vi "LtaExample.vi"() -> ()   [LabVIEW 2018]
uses:
  Comms_lib/CommsData.ctl
  <extravilib>/ChannelInstances/Tag-bool/Write With Abort.vi
  <extravilib>/ChannelInstances/Tag-bool/Read With Abort.vi
  <extravilib>/ChannelInstances/Tag-bool/Instantiate.vi
  <extravilib>/ChannelInstances/Tag-bool/EndpointRead.vi
  <vilib>/Utility/error.llb/Error Cluster From Error Code.vi
  <extravilib>/ChannelInstances/Tag-bool/Endpoint.vi
  <vilib>/ErrorRing/Error Ring.xnode
  Comms_lib/Comms.lvlib
  <extravilib>/ChannelInstances/Tag-bool.lvlib
  LV-PY_Lib/LV-PY.lvlib
panel:
  in  "MyCluster":T1
  out "Enum Out":enum16{"Foo", "Bar", "Do", "Rey", "Mi"}(ring)
  in  "btnRun":bool
  out "D":dbl
  in  "C":dbl=1.0
  in  "B":dbl=1.0
  in  "A":dbl=1.0
  in  "btnPlay":bool
  in  "Script":path=path "X:/Projects/PMUCal/LV_TestAutomation/Examples/example.py"
  out "Accepted?":bool
  in  "btnStop":bool
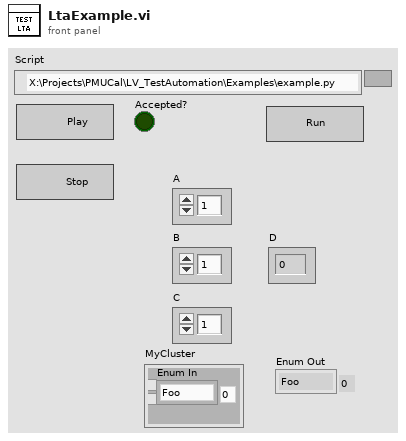
[diagram p1: front panel]
types:
  T1 = cluster{"Enum In":enum16{"Foo", "Bar", "Do", "Rey", "Mi"}}
  T2 = typedef "Comms.lvlib/CommsData.ctl" = cluster{"Command":string, "XMLData":string}
  T3 = typedef "Tag-bool.lvlib/))Channel.ctl" = refnum<queue>
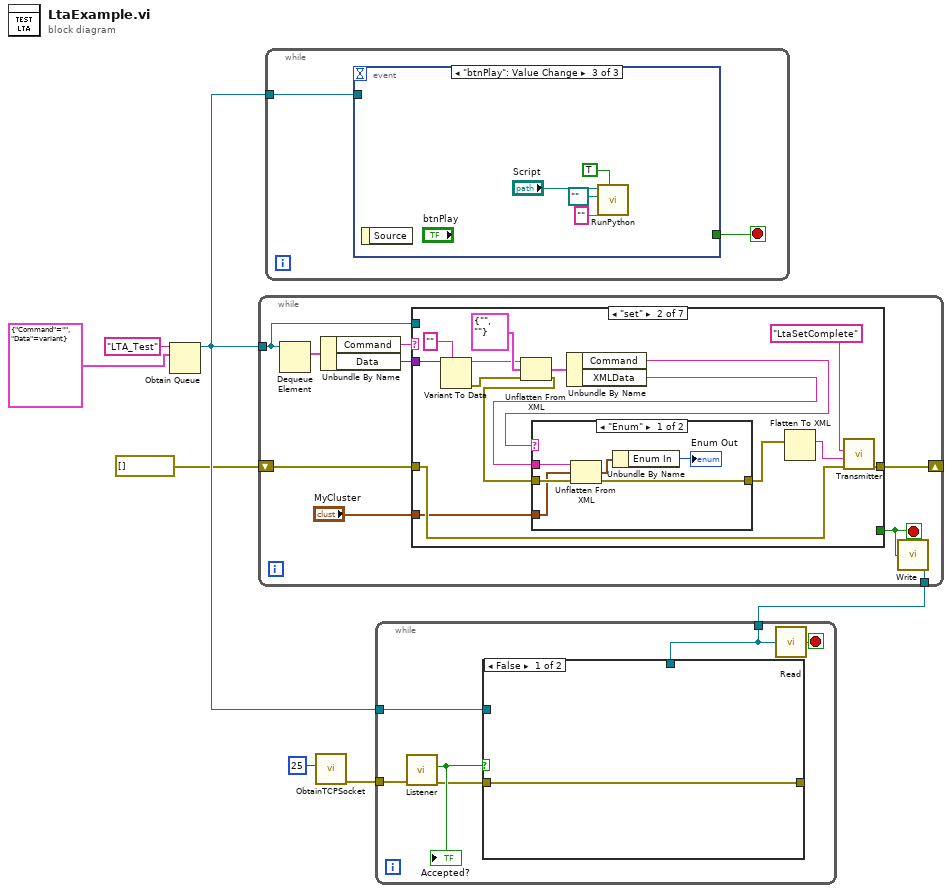
[diagram p0: block diagram]
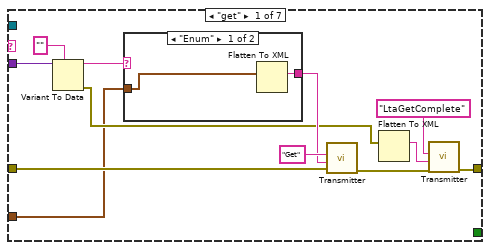
[diagram p2: hidden frame]
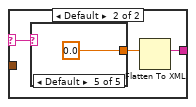
[diagram p3: hidden frame]
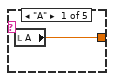
[diagram p4: hidden frame]
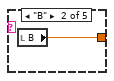
[diagram p5: hidden frame]
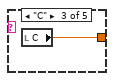
[diagram p6: hidden frame]
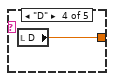
[diagram p7: hidden frame]
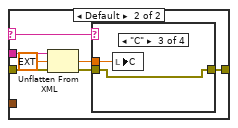
[diagram p8: hidden frame]
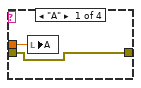
[diagram p9: hidden frame]
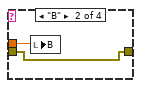
[diagram p10: hidden frame]
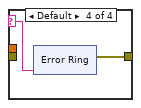
[diagram p11: hidden frame]
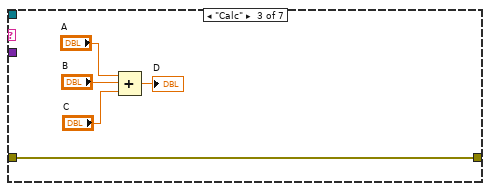
[diagram p12: hidden frame]
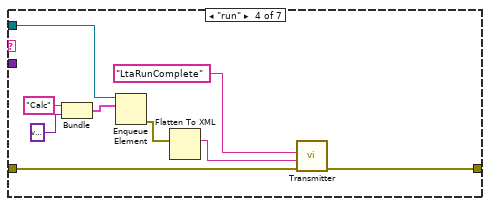
[diagram p13: hidden frame]
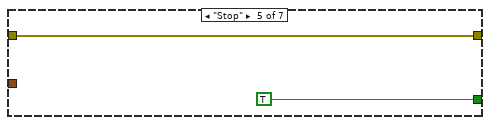
[diagram p14: hidden frame]
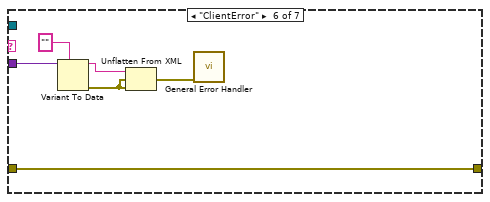
[diagram p15: hidden frame]
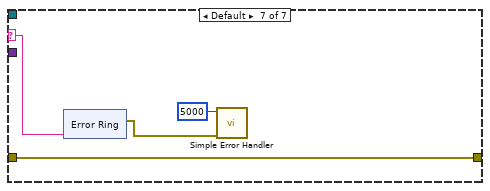
[diagram p16: hidden frame]
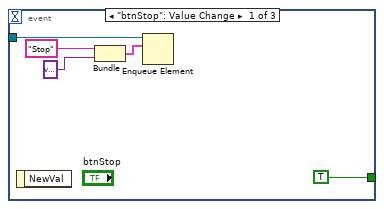
[diagram p17: hidden frame]
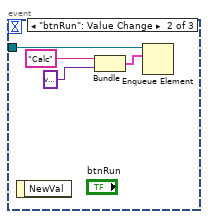
[diagram p18: hidden frame]
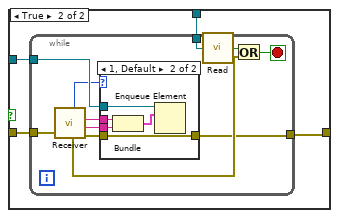
[diagram p19: hidden frame]
diagram:
  n1 = Obtain Queue(name (unnamed)="LTA_Test", element data type=cluster{"Command":string, "Data":variant} {"Command"="", "Data"=variant}) -> (queue out=w2:refnum<queue>)  [unwired: 3 in, 2 out]
  n2 = while {
    tunnel: [w12] -> w5
    tunnel: w2 -> [w11]
    shift-right: [w10] -> _
    shift-left: errorcluster[] [] ("ErrorArray") -> [w9]
    stop <- w13 stop-if-true
    n3 = Dequeue Element(queue=w11) -> (element=w16:cluster{"Command":string, "Data":variant})  [unwired: 2 in, 3 out]
    n4 = Unbundle By Name(w16) -> ("Command"=w15:string, "Data"=w14:variant)
    n5 = case shown="\"set\"" w15 {
      selector: w15 -> [_ _ _ _ _ _ w106]
      tunnel: w14 -> [w28 w53 _ _ _ w103 _]
      tunnel: [_ _ _ _ TRUE _ _] -> w13
      tunnel: w11 -> [_ _ _ w95 _ _ _]
      tunnel: [w22 w51 w82 w91 w96 w98 w104] -> w10
      tunnel: w9 -> [w24 w40 w82 w90 w96 w98 w104]
      tunnel: "MyCluster" -> [w17 w39 _ _ _ _ _]
      frame "get" {
        n6 = Variant To Data(type="", Variant=w28) -> (data=w26:string, error out=w19:errorcluster)  [unwired: 1 in]
        n7 = case shown="\"Enum\"" w26 {
          selector: w26 -> [_ w33]
          tunnel: [w30 w31] -> w20
          tunnel: w17 -> [w29 _]
          frame "Enum" {
            n8 = Flatten To XML(anything=w29) -> (xml string=w30:string)
          }
          frame Default {
            n9 = case shown="Default" w33 {
              tunnel: [w34 w35 w36 w37 0.0 ("D")] -> w32
              frame "A" {
                n10 = local read "A"() -> (w34:dbl)
              }
              frame "B" {
                n11 = local read "B"() -> (w35:dbl)
              }
              frame "C" {
                n12 = local read "C"() -> (w36:dbl)
              }
              frame "D" {
                n13 = local read "D"() -> (w37:dbl)
              }
              frame Default {
              }
            }
            n14 = Flatten To XML(anything=w32) -> (xml string=w31:string)
          }
        }
        n15 = call "Transmitter.vi"("ErrorArray"=w24, "XMLData"=w20, "Command"="Get") -> ("ErrorArray"=w23:errorcluster[])  [unwired: 7 in, 1 out]
        n16 = Flatten To XML(anything=w19) -> (xml string=w18:string)
        n17 = call "Transmitter.vi"("ErrorArray"=w23, "XMLData"=w18, "Command"="LtaGetComplete") -> ("ErrorArray"=w22:errorcluster[])  [unwired: 7 in, 1 out]
      }
      frame "set" {
        n18 = Variant To Data(type="", Variant=w53) -> (data=w47:string, error out=w46:errorcluster)  [unwired: 1 in]
        n19 = Unflatten From XML(xml string=w47, type=T2 {"Command"="", "XMLData"=""} ("CommsData"), error in (no error)=w46) -> (value=w45:T2, error out=w42:errorcluster)
        n20 = Unbundle By Name(w45) -> ("Command"=w44:string, "XMLData"=w43:string)
        n21 = case shown="\"Enum\"" w44 {
          selector: w44 -> [_ w65]
          tunnel: w43 -> [w59 w64]
          tunnel: w42 -> [w58 w63]
          tunnel: [w57 w60] -> w41
          tunnel: w39 -> [w56 _]
          frame "Enum" {
            n22 = Unflatten From XML(xml string=w59, type=w56, error in (no error)=w58) -> (value=w55:T1, error out=w57:errorcluster)
            n23 = Unbundle By Name(w55) -> ("Enum In"=→"Enum Out":enum16{"Foo", "Bar", "Do", "Rey", "Mi"})
          }
          frame Default {
            n24 = Unflatten From XML(xml string=w64, type=ext 0.0 ("D"), error in (no error)=w63) -> (value=w62:ext, error out=w61:errorcluster)
            n25 = case shown="\"C\"" w65 {
              selector: w65 -> [_ _ _ w74]
              tunnel: w62 -> [w68 w70 w72 _]
              tunnel: w61 -> [w67 w69 w71 _]
              tunnel: [w67 w69 w71 w73] -> w60
              frame "A" {
                n26 = local write "A"(w68) -> ()
              }
              frame "B" {
                n27 = local write "B"(w70) -> ()
              }
              frame "C" {
                n28 = local write "C"(w72) -> ()
              }
              frame Default {
                n29 = xnode ("Error Ring")("parameter 0"=w74) -> ("error out"=w73:errorcluster)
              }
            }
          }
        }
        n30 = Flatten To XML(anything=w41) -> (xml string=w49:string)
        n31 = call "Transmitter.vi"("ErrorArray"=w40, "XMLData"=w49, "Command"="LtaSetComplete") -> ("ErrorArray"=w51:errorcluster[])  [unwired: 7 in, 1 out]
      }
      frame "Calc" {
        n32 = Compound Arithmetic op=ADD("A", "B", "C") -> (→"D":dbl)
      }
      frame "run" {
        n33 = Bundle("Calc", variant) -> (w94:cluster{string, variant})  [unwired: 1 in]
        n34 = Enqueue Element(queue=w95, element=w94) -> (error out=w88:errorcluster)  [unwired: 2 in, 2 out]
        n35 = Flatten To XML(anything=w88) -> (xml string=w89:string)
        n36 = call "Transmitter.vi"("ErrorArray"=w90, "XMLData"=w89, "Command"="LtaRunComplete") -> ("ErrorArray"=w91:errorcluster[])  [unwired: 7 in, 1 out]
      }
      frame "Stop" {
      }
      frame "ClientError" {
        n37 = Variant To Data(type="", Variant=w103) -> (data=w100:string, error out=w101:errorcluster)  [unwired: 1 in]
        n38 = Unflatten From XML(xml string=w100, type=w101, error in (no error)=w101) -> (value=w99:errorcluster)  [unwired: 1 out]
        n39 = call <vilib>:"General Error Handler.vi"("error in (no error)"=w99) -> ()  [unwired: 10 in, 5 out]
      }
      frame Default {
        n40 = xnode "Error Ring"("parameter 0"=w106) -> ("error out"=w105:errorcluster)
        n41 = call <vilib>:"Simple Error Handler.vi"("error code (no error:0)"=5000, "error in (no error)"=w105) -> ()  [unwired: 3 in, 5 out]
      }
    }
    n42 = call <extravilib>:"Write.vi"("element"=w13) -> ("channel"=w12:T3)  [unwired: 1 out]
  }
  n43 = while {
    tunnel: w2 -> [w115]
    stop <- w116 stop-if-true
    n44 = event shown="[2] \"btnPlay\": Value Change" {
      selector: _ -> [_ _ _]
      dyn-events: _ -> [_ _ _]
      timeout: _ -> [_ _ _]
      tunnel: [TRUE _ _] -> w116
      tunnel: w115 -> [w120 w125 _]
      event "btnStop": Value Change {
        n45 = event-data() -> ()  [unwired: 1 in, 1 out]
        n46 = Bundle("Stop", variant) -> (w119:cluster{string, variant})  [unwired: 1 in]
        n47 = Enqueue Element(queue=w120, element=w119) -> ()  [unwired: 2 in, 3 out]
      }
      event "btnRun": Value Change {
        n48 = event-data() -> ()  [unwired: 1 in, 1 out]
        n49 = Bundle("Calc", variant) -> (w124:cluster{string, variant})  [unwired: 1 in]
        n50 = Enqueue Element(queue=w125, element=w124) -> ()  [unwired: 2 in, 3 out]
      }
      event "btnPlay": Value Change {
        n51 = event-data() -> ()  [unwired: 1 in, 1 out]
        n52 = call "RunPython.vi"("PathToScript"="Script", "PathToUserDir"=path "", "ScriptDir"="", "keep cmd window open (f)"=TRUE) -> ()  [unwired: 5 in, 2 out]
      }
    }
  }
  n53 = call "ObtainTCPSocket.vi"("timeout"=25) -> ("ErrorArray"=w6:errorcluster[])  [unwired: 9 in, 1 out]
  n54 = while {
    tunnel: w6 -> [w135]
    tunnel: w5 -> [w131]
    tunnel: w2 -> [w130]
    stop <- w134 stop-if-true
    n55 = call "Listener.vi"("ErrorArray"=w135) -> ("ErrorArray"=w132:errorcluster[], "Accepted?"=w133:bool)  [unwired: 9 in]
    "Accepted?" <- w133
    n56 = case shown="False" w133 {
      tunnel: w132 -> [w136 w140]
      tunnel: [w136 w138] -> _
      tunnel: w131 -> [_ w139]
      tunnel: w130 -> [_ w137]
      frame False {
      }
      frame True {
        n57 = while {
          tunnel: w140 -> [w151]
          tunnel: [w141] -> w138
          tunnel: w139 -> [w150]
          tunnel: w137 -> [w144]
          stop <- w148 stop-if-true
          n58 = call "Receiver.vi"("ErrorArray"=w151) -> ("ErrorArray"=w142:errorcluster[], "XMLData"=w145:string, "Command"=w146:string, "error out"=w147:errorcluster, "bytes_read"=w143:i32)  [unwired: 6 in]
          n59 = case shown="1, Default" w143 {
            tunnel: w146 -> [_ w156]
            tunnel: w145 -> [_ w155]
            tunnel: w144 -> [_ w154]
            tunnel: w142 -> [w152 w153]
            tunnel: [w152 w153] -> w141
            frame 0 {
            }
            frame 1, Default {
              n60 = Bundle("Command"=w156, "XMLData"=w155) -> (w157:cluster{"Command":string, "XMLData":string})  [unwired: 1 in]
              n61 = Enqueue Element(queue=w154, element=w157) -> ()  [unwired: 2 in, 3 out]
            }
          }
          n62 = call <extravilib>:"Read.vi"("channel"=w150) -> ("element"=w149:bool)  [unwired: 1 in, 1 out]
          n63 = Or(x=w149, y=w147) -> (x .or. y?=w148:bool)
        }
      }
    }
    n64 = call <extravilib>:"Read.vi"("channel"=w131) -> ("element"=w134:bool)  [unwired: 1 in, 1 out]
  }
